vi "add to memory format.vi"(8 "error in":errorcluster, 9 "CEF_serializable configuration in":refnum<class "CEF_serializable configuration.lvclass">, 10 "parent ID":string, 11 "memory hierarchy in":T1) -> (0 "error out":errorcluster, 3 "memory hierarchy out":T1)   [LabVIEW 2023, in "CEF.lvlib"]
doc: "Add an instance as the child of a given node in the object (unflattened) form of the hierarchyCopyright 2017 National Instruments Corporation\n\nLicensed under the Apache License, Version 2.0 (the \"License\"); you may not use this file except in compliance with the License. You may obtain a copy of the License at http://www.apache.org/licenses/LICENSE-2.0\nUnless required by applicable law or agreed to in writing, software distributed under the License is distributed on an \"AS IS\" BASIS, WITHOUT WARRANTIES OR CONDITIONS OF ANY KIND, either express or implied. See the License for the specific language governing permissions and limitations under the License."
uses:
  CEF.lvlib
  hierarchy repo/memory hierarchy.ctl
  hierarchy repo/full hierarchy.ctl
  hierarchy element.ctl
  serializable configuration/CEF_serializable configuration.lvclass
  serializable configuration/CEF_serializable configuration.lvclass/CEF_serializable configuration.ctl
  <vilib>/Utility/LVClass/Get LV Class Name.vi
  hierarchy repo/CEF_HierarchyRepo.lvclass
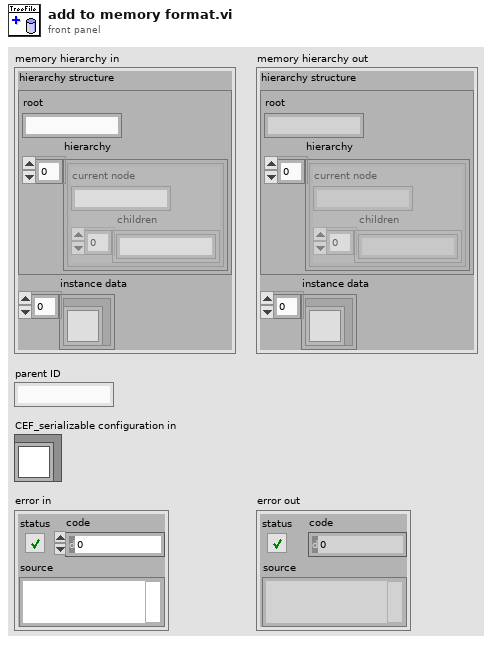
[diagram p1: front panel]
types:
  T1 = typedef "CEF.lvlib/CEF_HierarchyRepo.lvclass/memory hierarchy.ctl" = cluster{"hierarchy structure":T2, "instance data":refnum<class "CEF_serializable configuration.lvclass">[]}
  T2 = typedef "CEF.lvlib/CEF_HierarchyRepo.lvclass/full hierarchy.ctl" = cluster{"root":string, "hierarchy":T3[]}
  T3 = typedef "CEF.lvlib/hierarchy element.ctl" = cluster{"current node":string, "children":string[]}
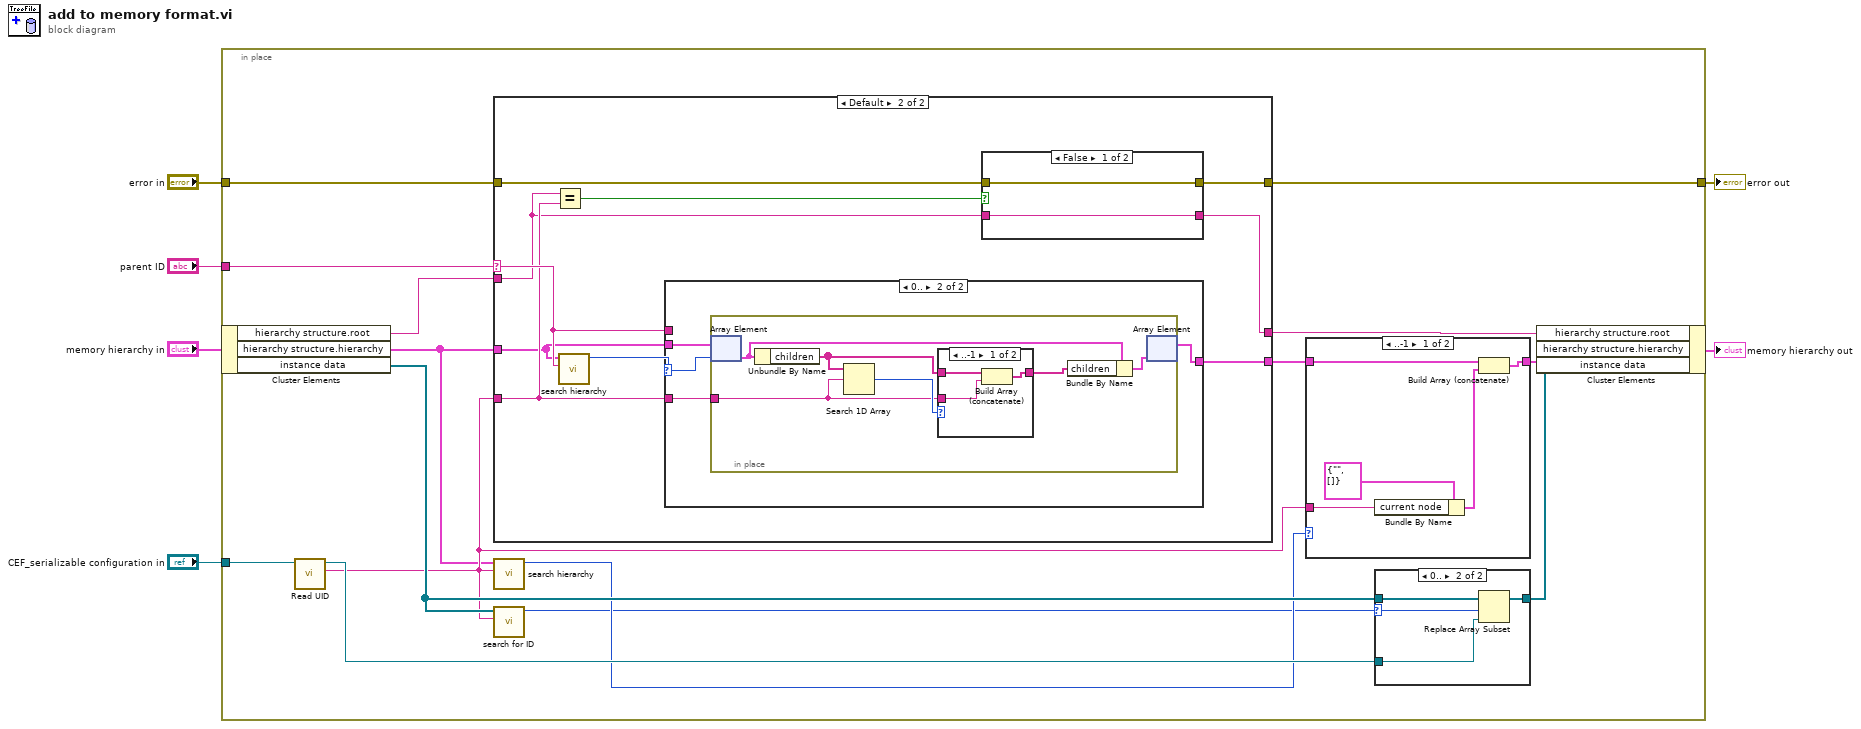
[diagram p0: block diagram]
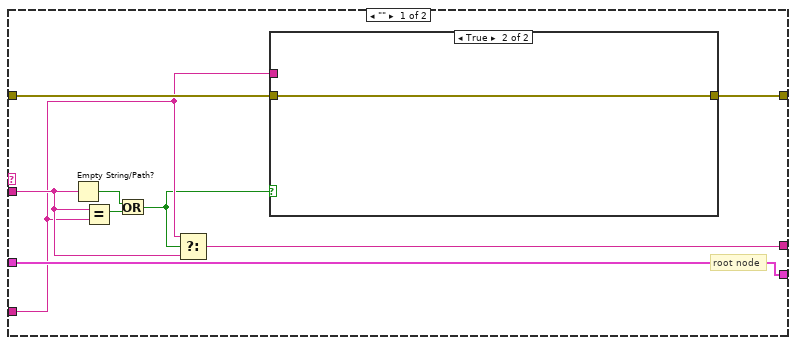
[diagram p2: hidden frame]
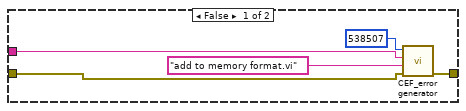
[diagram p3: hidden frame]
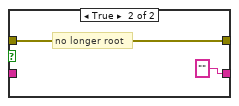
[diagram p4: hidden frame]
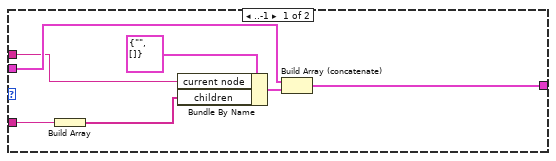
[diagram p5: hidden frame]
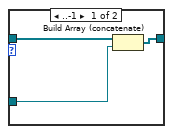
[diagram p8: hidden frame]
diagram:
  n1 = in-place {
    in-place-border: "CEF_serializable configuration in" -> [w21]
    in-place-border: "parent ID" -> [w15]
    in-place-border: "error in" -> [w11]
    in-place-border: [w10] -> w1
    n2 = in-place-cluster #1("memory hierarchy in") -> ("hierarchy structure.root"=w14:string, "hierarchy structure.hierarchy"=w7:T3[], "instance data"=w19:refnum<class "CEF_serializable configuration.lvclass">[])
    n3 = call "Read UID.vi"("CEF_Configuration in"=w21) -> ("instance id"=w12:string, "CEF_Configuration out"=w18:refnum<class "CEF_serializable configuration.lvclass">)  [unwired: 8 in, 1 out]
    n4 = case shown="Default" w15 {
      selector: w15 -> [_ w45]
      tunnel: w7 -> [w30 w37]
      tunnel: [w30 w46] -> w17
      tunnel: w12 -> [w23 w44]
      tunnel: w14 -> [w24 w41]
      tunnel: [w29 w42] -> w13
      tunnel: w11 -> [w28 w39]
      tunnel: [w27 w40] -> w10
      frame "" {
        # "root node"
        n5 = Empty String/Path?(string/path=w24) -> (empty?=w25:bool)
        n6 = Equal?(x=w24, y=w23) -> (x = y?=w26:bool)
        n7 = Or(x=w25, y=w26) -> (x .or. y?=w22:bool)
        n8 = Select(t=w23, s=w22, f=w24) -> (s? t:f=w29:string)
        n9 = case shown="True" w22 {
          tunnel: w28 -> [w35 w36]
          tunnel: [w34 w36] -> w27
          tunnel: w23 -> [w32 _]
          frame False {
            n10 = call "CEF_error generator.vi"("error in"=w35, "source"="add to memory format.vi", "append error message"=w32, "error code (0)"=538507) -> ("error out"=w34:errorcluster)  [unwired: 5 in]
          }
          frame True {
          }
        }
      }
      frame Default {
        n11 = Equal?(x=w41, y=w44) -> (x = y?=w43:bool)
        n12 = call "search hierarchy.vi"("ID"=w45, "hierarchy"=w37) -> ("index"=w38:i32)  [unwired: 9 in]
        n13 = case shown="0.." w38 {
          selector: w38 -> [_ w58]
          tunnel: w37 -> [w55 w61]
          tunnel: [w52 w60] -> w46
          tunnel: w44 -> [w54 w59]
          tunnel: w45 -> [w51 _]
          frame ..-1 {
            n14 = Build Array(w54) -> (w53:string[])
            n15 = Bundle By Name(cluster=T3 {"current node"="", "children"=[]} ("hierarchy"), "current node"=w51, "children"=w53) -> (w57:T3)
            n16 = Build Array (concatenate)(w55, w57) -> (w52:T3[])
          }
          frame 0.. {
            n17 = in-place {
              in-place-border: w59 -> [w63]
              n18 = in-place-array #2(w61, w58) -> (w67:T3)
              n19 = Unbundle By Name(w67) -> ("children"=w64:string[])
              n20 = Search 1D Array(1D array=w64, element=w63) -> (index of element=w65:i32)  [unwired: 1 in]
              n21 = case shown="..-1" w65 {
                tunnel: w64 -> [w70 w71]
                tunnel: w63 -> [w69 _]
                tunnel: [w68 w71] -> w62
                frame ..-1 {
                  n22 = Build Array (concatenate)(w70, w69) -> (w68:string[])
                }
                frame 0.. {
                }
              }
              n23 = Bundle By Name(cluster=w67, "children"=w62) -> (w66:T3)
              n24 = in-place-array #2(w66) -> (w60:T3[])  [unwired: 1 out]
            }
          }
        }
        n25 = case shown="False" w43 {
          tunnel: [w48 "" ("root")] -> w42
          tunnel: w41 -> [w48 _]
          tunnel: [w47 w50] -> w40
          tunnel: w39 -> [w47 w50]
          frame False {
          }
          frame True {
            # "no longer root"
          }
        }
      }
    }
    n26 = call "search hierarchy.vi"("ID"=w12, "hierarchy"=w7) -> ("index"=w9:i32)  [unwired: 9 in]
    n27 = call "search for ID.vi"("instance id"=w12, "instance data"=w19) -> ("index"=w8:i32)  [unwired: 9 in]
    n28 = case shown="..-1" w9 {
      tunnel: w17 -> [w76 w77]
      tunnel: [w75 w77] -> w16
      tunnel: w12 -> [w73 _]
      frame ..-1 {
        n29 = Bundle By Name(cluster=T3 {"current node"="", "children"=[]} ("hierarchy"), "current node"=w73) -> (w72:T3)
        n30 = Build Array (concatenate)(w76, w72) -> (w75:T3[])
      }
      frame 0.. {
      }
    }
    n31 = case shown="0.." w8 {
      selector: w8 -> [_ w81]
      tunnel: [w79 w83] -> w20
      tunnel: w19 -> [w78 w84]
      tunnel: w18 -> [w80 w82]
      frame ..-1 {
        n32 = Build Array (concatenate)(w78, w80) -> (w79:refnum<class "CEF_serializable configuration.lvclass">[])
      }
      frame 0.. {
        n33 = Replace Array Subset(array=w84, new element=w82, index=w81) -> (w83:refnum<class "CEF_serializable configuration.lvclass">[])
      }
    }
    n34 = in-place-cluster #1("hierarchy structure.root"=w13, "hierarchy structure.hierarchy"=w16, "instance data"=w20) -> (→"memory hierarchy out":T1)
  }
  "error out" <- w1
